vi "诊断标定4.vi"(8 "CAN端口":u16(ring), 9 "设备索引号":u16(ring), 10 "CAN卡类型":u32(ring)=4) -> ()   [LabVIEW 2013] (continued)
                    n1590 = Increment(x=w2571) -> (x+1=w2730:i32)
                    n1591 = global write "读配置文件全局.vi" "从板个数"(w2571) -> ()
                    n1592 = local write "从板个数"(w2571) -> ()
                    n1593 = Index Array(array=w2594, index #1=4 ("索引"), index #2=5 ("索引"), index #3=6 ("索引")) -> (element #1=w2738:string, element #2=w2737:string, element #3=w2736:string)
                    n1594 = Index Array(array=w2747) -> (element #1=w2745:dbl, element #2=w2744:dbl, element #3=w2743:dbl, element #4=w2742:dbl)  [unwired: 4 in]
                    n1595 = Array Subset(array=w2598, index=w2723, length=w2731) -> (w2715:string[])
                    n1596 = Array Subset(array=w2598, index=w2722, length=w2730) -> (w2713:string[])
                    n1597 = Array Subset(array=w2598, index=w2721, length=w2729) -> (w2712:string[])
                    n1598 = Array Subset(array=w2598, index=w2720, length=w2716) -> (w2711:string[])
                    n1599 = Array Subset(array=w2598, index=w2719, length=20 ("长度")) -> (w2710:string[])
                    n1600 = Array Subset(array=w2598, index=w2718, length=w2717) -> (w2714:string[])
                    n1601 = control-ref of="项目信息2"() -> (w2750:refnum<vi>)
                    n1602 = Insert Into Array(array=w2715, new element #1=w2714, new element #2=w2713, new element #3=w2712, new element #4=w2711, new element #5=w2710) -> (w2568:string[])  [unwired: 1 in]
                    n1603 = property class="Clust (严格)"(reference=w2750) -> (reference out=w2748:refnum<vi>, "Value"=w2749:T8)  [unwired: 1 in, 1 out]
                    n1604 = Array Subset(array=w2602, index=w2723, length=w2716) -> (w2584:string[])
                    n1605 = Array Subset(array=w2602, index=w2722, length=w2716) -> (w2582:string[])
                    n1606 = Array Subset(array=w2602, index=w2721, length=w2716) -> (w2581:string[])
                    n1607 = Array Subset(array=w2602, index=w2720) -> (w2580:string[])  [unwired: 1 in]
                    n1608 = Array Subset(array=w2602, index=w2719, length=w2717) -> (w2579:string[])
                    n1609 = Array Subset(array=w2602, index=w2718, length=w2717) -> (w2583:string[])
                    n1610 = global write "读配置文件全局.vi" "表格输入"(w2568) -> ()
                    n1611 = Bundle(cluster=w2749, "电池额定容量(A)"=w2745, "使用者"=w2735, "电池实际容量(A)"=w2744, "车架(牌)号"=w2737, "配置文件版本"=w2736, "SOH(%)"=w2742, "SOC(%)"=w2743, "产品编号"=w2738) -> (w2569:T8)  [unwired: 1 in]
                    n1612 = Multiply(x=w2571, y=4) -> (x*y=w2575:i32)
                    n1613 = Insert Into Array(array=w2584, new element #1=w2583, new element #2=w2582, new element #3=w2581, new element #4=w2580, new element #5=w2579) -> (w2578:string[])  [unwired: 1 in]
                    n1614 = Add(x=w2575, y=44) -> (x+y=w2573:i32)
                    n1615 = property class="Clust (严格)"(reference=w2748, "Value"=w2569) -> ()  [unwired: 1 in, 2 out]
                    n1616 = global write "读配置文件全局.vi" "项目信息"(w2569) -> ()
                    n1617 = Array Subset(array=w2578, index=0 ("索引"), length=w2573) -> (w2577:string[])
                    n1618 = Build Array(w2577, w2568) -> (w2709:string[][])
                    n1619 = Transpose 2D Array(2D array=w2709) -> (transposed array=w2570:string[][])
                    n1620 = local write "项目信息"(w2570) -> ()
                    n1621 = Array Subset(array=w2595, index=w2627, length=15 ("长度")) -> (w2559:string[])
                    n1622 = Array Subset(array=w2595, index=w2630, length=14 ("长度")) -> (w2635:string[])
                    n1623 = Delete From Array(array=w2559, length=4 ("长度"), index=6 ("索引")) -> (deleted portion=w2621:string[], array with subset deleted=w2620:string[])
                    n1624 = for {
                      tunnel: w2635 -> [w2763] mode=indexing
                      tunnel: [w2762] -> w2634 mode=indexing
                      n1625 = Fract/Exp String To Number(string=w2763) -> (number=w2762:dbl)  [unwired: 3 in, 1 out]
                    }
                    n1626 = for {
                      tunnel: w2620 -> [w2761] mode=indexing
                      tunnel: [w2760] -> w2619 mode=indexing
                      n1627 = Fract/Exp String To Number(string=w2761) -> (number=w2760:dbl)  [unwired: 3 in, 1 out]
                    }
                    n1628 = Array Subset(array=w2595, index=w2639, length=51 ("长度")) -> (w2708:string[])
                    n1629 = for {
                      tunnel: w2708 -> [w2765] mode=indexing
                      tunnel: [w2764] -> w2707 mode=indexing
                      n1630 = Fract/Exp String To Number(string=w2765) -> (number=w2764:dbl)  [unwired: 3 in, 1 out]
                    }
                    n1631 = Index Array(array=w2619) -> (element #1=w2614:dbl, element #2=w2613:dbl, element #3=w2612:dbl, element #4=w2611:dbl, element #5=w2610:dbl, element #6=w2609:dbl, element #7=w2608:dbl, element #8=w2607:dbl, element #9=w2606:dbl, element #10=w2605:dbl, element #11=w2604:dbl)  [unwired: 11 in]
                    n1632 = Delete From Array(array=w2634, length=7 ("长度"), index=0 ("索引")) -> (deleted portion=w2564:dbl[], array with subset deleted=w2632:dbl[])
                    n1633 = Delete From Array(array=w2707, length=17 ("长度"), index=0 ("索引")) -> (deleted portion=w2561:dbl[], array with subset deleted=w2704:dbl[])
                    n1634 = global write "读配置文件全局.vi" "加热控制参数"(w2564) -> ()
                    n1635 = Array To Cluster(array=w2564) -> (cluster=w2633:T23)
                    n1636 = Index Array(array=w2632) -> (element #1=w2592:dbl, element #2=w2591:dbl, element #3=w2590:dbl, element #4=w2589:dbl, element #5=w2588:dbl, element #6=w2587:dbl, element #7=w2586:dbl, element #8=w2585:dbl)  [unwired: 8 in]
                    n1637 = Delete From Array(array=w2704, length=17 ("长度"), index=0 ("索引")) -> (deleted portion=w2560:dbl[], array with subset deleted=w2557:dbl[])
                    n1638 = Index Array(array=w2621) -> (element #1=w2618:string, element #2=w2617:string, element #3=w2615:string, element #4=w2616:string)  [unwired: 4 in]
                    n1639 = local write "加热控制参数"(w2633) -> ()
                    n1640 = global write "读配置文件全局.vi" "一级故障"(w2561) -> ()
                    n1641 = local read "一级故障 5"() -> (w2593:T11)
                    n1642 = global write "读配置文件全局.vi" "二级故障"(w2560) -> ()
                    n1643 = control-ref of="电池信息"() -> (w2625:refnum<vi>)
                    n1644 = property class="Clust (严格)"(reference=w2625) -> (reference out=w2626:refnum<vi>, "Value"=w2624:T12)  [unwired: 1 in, 1 out]
                    n1645 = global write "读配置文件全局.vi" "三级故障"(w2557) -> ()
                    n1646 = Bundle(cluster=w2593, "最大允许单体电压"=w2592, "最大允许总电压"=w2588, "最小允许单体电压"=w2591, "最大允许充电电流"=w2590, "最小允许充电电流"=w2589, "最大允许充电温度"=w2587, "最小允许充电温度"=w2586, "电流步长"=w2585) -> (w2563:T11)
                    n1647 = Bundle(cluster=w2624, "电池串联"=w2614, "电池并联"=w2613, "累计放电总安时"=w2607, "电池包额定容量"=w2612, "电池包额定能量"=w2611, "电池包额定总电压"=w2610, "累计充电总安时"=w2608, "电池充满次数"=w2605, "电池放空次数"=w2606, "电池充电次数"=w2604, "电池生产日期"=w2615, "电池厂家"=w2618, "电池类型"=w2617, "电池包组号"=w2616, "实际容量"=w2609) -> (w2558:T12)  [unwired: 2 in]
                    n1648 = Cluster To Array(cluster=w2563) -> (array=w2562:dbl[])
                    n1649 = local write "一级故障 5"(w2563) -> ()
                    n1650 = global write "读配置文件全局.vi" "充电控制参数"(w2562) -> ()
                    n1651 = property class="Clust (严格)"(reference=w2626, "Value"=w2558) -> ()  [unwired: 1 in, 2 out]
                    n1652 = Index Array(array=w2561) -> (element #1=w2697:dbl, element #2=w2696:dbl, element #3=w2695:dbl, element #4=w2694:dbl, element #5=w2693:dbl, element #6=w2692:dbl, element #7=w2691:dbl, element #8=w2690:dbl, element #9=w2689:dbl, element #10=w2688:dbl, element #11=w2687:dbl, element #12=w2686:dbl, element #13=w2685:dbl, element #14=w2684:dbl, element #15=w2683:dbl, element #16=w2682:dbl, element #17=w2681:dbl)  [unwired: 17 in]
                    n1653 = global write "读配置文件全局.vi" "电池信息"(w2558) -> ()
                    n1654 = Index Array(array=w2560) -> (element #1=w2664:dbl, element #2=w2665:dbl, element #3=w2666:dbl, element #4=w2667:dbl, element #5=w2668:dbl, element #6=w2669:dbl, element #7=w2670:dbl, element #8=w2671:dbl, element #9=w2672:dbl, element #10=w2673:dbl, element #11=w2674:dbl, element #12=w2675:dbl, element #13=w2676:dbl, element #14=w2677:dbl, element #15=w2678:dbl, element #16=w2679:dbl, element #17=w2680:dbl)  [unwired: 17 in]
                    n1655 = Index Array(array=w2557) -> (element #1=w2659:dbl, element #2=w2658:dbl, element #3=w2657:dbl, element #4=w2656:dbl, element #5=w2655:dbl, element #6=w2654:dbl, element #7=w2653:dbl, element #8=w2652:dbl, element #9=w2651:dbl, element #10=w2650:dbl, element #11=w2649:dbl, element #12=w2648:dbl, element #13=w2647:dbl, element #14=w2646:dbl, element #15=w2645:dbl, element #16=w2644:dbl, element #17=w2643:dbl)  [unwired: 17 in]
                    n1656 = control-ref of="一级故障 3"() -> (w2642:refnum<vi>)
                    n1657 = control-ref of="一级故障 2"() -> (w2661:refnum<vi>)
                    n1658 = property class="Clust (严格)"(reference=w2661) -> (reference out=w2663:refnum<vi>, "Value"=w2662:T9)  [unwired: 1 in, 1 out]
                    n1659 = property class="Clust (严格)"(reference=w2642) -> (reference out=w2641:refnum<vi>, "Value"=w2660:T9)  [unwired: 1 in, 1 out]
                    n1660 = Bundle(cluster=w2662, "总电压过高"=w2664, "整组电压不均衡"=w2668, "SOC过高"=w2676, "单体电压过高"=w2672, "总电压过低"=w2665, "温度过高"=w2666, "温度过低"=w2667, "单组电压不均衡"=w2669, "整组温度不均衡"=w2670, "单组温度不均衡"=w2671, "单体电压过低"=w2673, "充电电流过高"=w2674, "放电电流过高"=w2675, "SOC过低"=w2677, "内阻过大"=w2678, "极柱温度过高"=w2679, "SOH过低"=w2680) -> (w2566:T9)
                    n1661 = Bundle(cluster=w2660, "总电压过高"=w2659, "整组电压不均衡"=w2655, "SOC过高"=w2647, "单体电压过高"=w2651, "总电压过低"=w2658, "温度过高"=w2657, "温度过低"=w2656, "单组电压不均衡"=w2654, "整组温度不均衡"=w2653, "单组温度不均衡"=w2652, "单体电压过低"=w2650, "充电电流过高"=w2649, "放电电流过高"=w2648, "SOC过低"=w2646, "内阻过大"=w2645, "极柱温度过高"=w2644, "SOH过低"=w2643) -> (w2565:T9)
                    n1662 = control-ref of="一级故障"() -> (w2700:refnum<vi>)
                    n1663 = property class="Clust (严格)"(reference=w2700) -> (reference out=w2698:refnum<vi>, "Value"=w2699:T9)  [unwired: 1 in, 1 out]
                    n1664 = Bundle(cluster=w2699, "总电压过高"=w2697, "整组电压不均衡"=w2693, "SOC过高"=w2685, "单体电压过高"=w2689, "总电压过低"=w2696, "温度过高"=w2695, "温度过低"=w2694, "单组电压不均衡"=w2692, "整组温度不均衡"=w2691, "单组温度不均衡"=w2690, "单体电压过低"=w2688, "充电电流过高"=w2687, "放电电流过高"=w2686, "SOC过低"=w2684, "内阻过大"=w2683, "极柱温度过高"=w2682, "SOH过低"=w2681) -> (w2567:T9)
                    n1665 = property class="Clust (严格)"(reference=w2698, "Value"=w2567) -> ()  [unwired: 1 in, 2 out]
                    n1666 = property class="Clust (严格)"(reference=w2663, "Value"=w2566) -> ()  [unwired: 1 in, 2 out]
                    n1667 = property class="Clust (严格)"(reference=w2641, "Value"=w2565) -> ()  [unwired: 1 in, 2 out]
                  }
                  frame #2 {
                    (unwired) 2 ("长度")
                    w2808 = 1 ("索引")
                    n1668 = call <vilib>:"Get Section Names.vi"("refnum"=w2824) -> ("section names"=w2825:string[], "refnum out"=w2829:T22)  [unwired: 8 in, 1 out]
                    n1669 = local read "从板板号"() -> (w2806:u8)
                    n1670 = Delete From Array(array=w2825, length=2 ("长度"), index=0 ("索引")) -> (array with subset deleted=w2828:string[])  [unwired: 1 out]
                    n1671 = for {
                      tunnel: w2828 -> [w2843] mode=indexing
                      tunnel: w2829 -> [w2844]
                      tunnel: [w2836] -> w2805 mode=indexing
                      tunnel: [w2835] -> w2794
                      n1672 = call <vilib>:"Get Key Names.vi"("section"=w2843, "refnum"=w2844) -> ("key names"=w2835:string[], "refnum out"=w2842:T22)  [unwired: 6 in, 2 out]
                      n1673 = for {
                        tunnel: w2835 -> [w2848] mode=indexing
                        tunnel: w2843 -> [w2847]
                        tunnel: w2842 -> [w2846]
                        tunnel: [w2845] -> w2836 mode=indexing
                        n1674 = call-poly <vilib>:"Read Key.vi"("section"=w2847, "key"=w2848, "refnum"=w2846) -> ("value"=w2845:string)  [unwired: 5 in, 3 out]
                      }
                      n1675 = Index Array(array=w2836, index=0 ("索引")) -> (element=w2839:string)
                      n1676 = local read "输出数组"() -> (w2840:string[][])
                      n1677 = Decimal String To Number(string=w2839) -> (number=w2838:i32)  [unwired: 2 in, 1 out]
                      n1678 = Decrement(x=w2838) -> (x-1=w2834:i32)
                      n1679 = Replace Array Subset(array=w2840, new element=w2836, index (col)=w2834) -> (w2837:string[][])  [unwired: 1 in]
                      n1680 = local write "输出数组"(w2837) -> ()
                    }
                    "key names" <- w2794
                    n1681 = Decrement(x=w2806) -> (x-1=w2823:u8)
                    n1682 = Index Array(array=w2805, index (row)=w2823) -> (element=w2778:string[])  [unwired: 1 in]
                    n1683 = Search 1D Array(1D array=w2794, element="风机开启温度" ("元素")) -> (index of element=w2811:i32)  [unwired: 1 in]
                    n1684 = Search 1D Array(1D array=w2794, element="电压过高一级" ("元素"), start index (0)=w2811) -> (index of element=w2813:i32)
                    n1685 = Decrement(x=w2811) -> (x-1=w2809:i32)
                    n1686 = Array Subset(array=w2778, index=w2808, length=w2809) -> (w2784:string[])
                    n1687 = Array Subset(array=w2778, index=w2813, length=21 ("长度")) -> (w2821:string[])
                    n1688 = Array Subset(array=w2794, index=w2808, length=w2809) -> (w2783:string[])
                    n1689 = Array Subset(array=w2778, index=w2811, length=7 ("长度")) -> (w2815:string[])
                    n1690 = for {
                      tunnel: w2821 -> [w2831] mode=indexing
                      tunnel: [w2830] -> w2822 mode=indexing
                      n1691 = Fract/Exp String To Number(string=w2831) -> (number=w2830:dbl)  [unwired: 3 in, 1 out]
                    }
                    n1692 = for {
                      tunnel: w2815 -> [w2833] mode=indexing
                      tunnel: [w2832] -> w2780 mode=indexing
                      n1693 = Fract/Exp String To Number(string=w2833) -> (number=w2832:dbl)  [unwired: 3 in, 1 out]
                    }
                    n1694 = Index Array(array=w2778, index=0 ("索引")) -> (element=w2776:string)
                    n1695 = Decimal String To Number(string=w2776) -> (number=w2775:i32)  [unwired: 2 in, 1 out]
                    n1696 = Delete From Array(array=w2822, length=7 ("长度"), index=0 ("索引")) -> (deleted portion=w2782:dbl[], array with subset deleted=w2818:dbl[])
                    n1697 = Array To Cluster(array=w2780) -> (cluster=w2804:T23)
                    n1698 = global write "读配置文件全局2.vi" "加热控制参数"(w2780) -> ()
                    n1699 = global write "读配置文件全局2.vi" "从板板号"(w2775) -> ()
                    n1700 = Delete From Array(array=w2818, length=7 ("长度"), index=0 ("索引")) -> (deleted portion=w2773:dbl[], array with subset deleted=w2774:dbl[])
                    n1701 = local write "加热控制参数"(w2804) -> ()
                    n1702 = Array To Cluster(array=w2782) -> (cluster=w2787:T23)
                    n1703 = Array To Cluster(array=w2774) -> (cluster=w2785:T23)
                    n1704 = Array To Cluster(array=w2773) -> (cluster=w2786:T23)
                    n1705 = global write "读配置文件全局2.vi" "三级故障阀值"(w2774) -> ()
                    n1706 = global write "读配置文件全局2.vi" "一级故障阀值"(w2782) -> ()
                    n1707 = global write "读配置文件全局2.vi" "二级故障阀值"(w2773) -> ()
                    n1708 = local write "一级故障 6"(w2787) -> ()
                    n1709 = local write "一级故障 8"(w2785) -> ()
                    n1710 = local write "一级故障 7"(w2786) -> ()
                    n1711 = Search 1D Array(1D array=w2783, element="温度个数" ("元素")) -> (index of element=w2798:i32)  [unwired: 1 in]
                    n1712 = Search 1D Array(1D array=w2783, element="第一个保险通道" ("元素")) -> (index of element=w2797:i32)  [unwired: 1 in]
                    n1713 = Search 1D Array(1D array=w2783, element="电压个数" ("元素")) -> ()  [unwired: 1 in, 1 out]
                    n1714 = Search 1D Array(1D array=w2783, element="第1通道电压个数" ("元素")) -> (index of element=w2796:i32)  [unwired: 1 in]
                    n1715 = Array Subset(array=w2784, length=2 ("长度")) -> (w2792:string[])  [unwired: 1 in]
                    n1716 = Array Subset(array=w2784, index=w2798) -> (w2790:string[])  [unwired: 1 in]
                    n1717 = Array Subset(array=w2784, index=w2797, length=20 ("长度")) -> (w2789:string[])
                    n1718 = Array Subset(array=w2784, index=w2796, length=20 ("长度")) -> (w2791:string[])
                    n1719 = Insert Into Array(array=w2792, new element #1=w2791, new element #2=w2790, new element #3=w2789) -> (w2779:string[])  [unwired: 1 in]
                    n1720 = Build Array(string[] ["电压个数", "电压起始值", "第1通道电压个数", "第2通道电压个数", "第3通道电压个数", "第4通道电压个数", "第5通道电压个数", "第6通道电压个数", "第7通道电压个数", "第8通道电压个数", "第9通道电压个数", "第10通道电压个数", "第11通道电压个数", "第12通道电压个数", "第13通道电压个数", "第14通道电压个数", "第15通道电压个数", "第16通道电压个数", "第17通道电压个数", "第18通道电压个数", "第19通道电压个数", "第20通道电压个数", "温度个数", "温度起始值", "第一个保险通道", "第一个保险位置", "第二个保险通道", "第二个保险位置", "第三个保险通道", "第三个保险位置", "第四个保险通道", "第四个保险位置", "第五个保险通道", "第五个保险位置", "第六个保险通道", "第六个保险位置", "第七个保险通道", "第七个保险位置", "第八个保险通道", "第八个保险位置", "第九个保险通道", "第九个保险位置", "第十个保险通道", "第十个保险位置"], w2779) -> (w2788:string[][])
                    n1721 = global write "读配置文件全局2.vi" "表格"(w2779) -> ()
                    n1722 = Transpose 2D Array(2D array=w2788) -> (transposed array=w2781:string[][])
                    n1723 = local write "项目信息 2"(w2781) -> ()
                  }
                  frame #3 {
                    n1724 = call <vilib>:"Unset Busy.vi"() -> ()  [unwired: 11 in, 1 out]
                    n1725 = Build Array("读取完成") -> (w2852:string[])
                    n1726 = property on="全部写入" class="Bool (严格)"("DisabledEnum"=0) -> ()  [unwired: 2 in, 2 out]
                    n1727 = call "表格编辑.vi"("新元素/子数组"=w2852, "活动单元格:单元格背景色"=u32 6618880, "MCListbox引用句柄"=w2849) -> ()  [unwired: 9 out]
                  }
                }
              }
            }
          }
        }
      }
      frame Error {
      }
    }
  }
  n1728 = while {
    tunnel: w17 -> [w2874]
    tunnel: w16 -> [w2873]
    tunnel: [w2872] -> w15
    tunnel: [w2871] -> w14
    stop <- w2870 stop-if-true
    n1729 = event shown="[33] \"风机继电器\": 值改变" {
      selector: _ -> [_ _ _ _ _ _ _ _ _ _ _ _ _ _ _ _ _ _ _ _ _ _ _ _ _ _ _ _ _ _ _ _ _ _ _ _ _ _ _ _ _ _ _ _ _ _ _ _ _ _ _]
      dyn-events: _ -> [_ _ _ _ _ _ _ _ _ _ _ _ _ _ _ _ _ _ _ _ _ _ _ _ _ _ _ _ _ _ _ _ _ _ _ _ _ _ _ _ _ _ _ _ _ _ _ _ _ _ _]
      timeout: 200 -> [_ _ _ _ _ _ _ _ _ _ _ _ _ _ _ _ _ _ _ _ _ _ _ _ _ _ _ _ _ _ _ _ _ _ _ _ _ _ _ _ _ _ _ _ _ _ _ _ _ _ _]
      tunnel: [_ w2877 w2905 _ _ _ _ _ _ _ _ _ _ _ _ _ _ _ _ _ _ _ _ _ _ _ _ _ _ _ _ _ _ _ _ _ _ _ _ _ _ _ _ _ _ _ _ _ _ _ _] -> w2869
      tunnel: w2874 -> [w2876 w2880 w2904 w2926 w2932 w2938 w2944 w2950 w2956 w2962 w2968 w2974 w2980 w2986 w3002 w3509 w3761 w3786 w3812 w3896 w3969 w3982 w3992 w4035 _ _ w4083 w4149 w4215 w4281 w4347 w4413 w4479 w4546 w4613 w4679 w4745 w4814 w4825 w4863 w4902 w4941 w4980 w5017 w5077 w5115 w5154 w5190 w5263 w5301 w5339]
      tunnel: w2873 -> [w2875 w2879 w2903 w2925 w2931 w2937 w2943 w2949 w2955 w2961 w2967 w2973 w2979 w2985 w3001 w3508 w3760 w3785 w3811 w3895 w3967 w3980 w3991 w4034 _ _ w4082 w4148 w4214 w4280 w4346 w4412 w4478 w4545 w4612 w4678 w4744 w4812 w4824 w4862 w4901 w4940 w4979 w5016 w5076 w5114 w5153 w5189 w5262 w5300 w5338]
      tunnel: [w2876 w2880 w2904 w2926 w2932 w2938 w2944 w2950 w2956 w2962 w2968 w2974 w2980 w2986 w3002 w3509 w3761 w3786 w3812 w3896 w3968 w3981 w3992 w4035 _ _ w4083 w4149 w4215 w4281 w4347 w4413 w4479 w4546 w4613 w4679 w4745 w4813 w4823 w4861 w4900 w4939 w4978 w5017 w5075 w5113 w5152 w5188 w5261 w5299 w5337] -> w2872
      tunnel: [w2875 w2879 w2903 w2925 w2931 w2937 w2943 w2949 w2955 w2961 w2967 w2973 w2979 w2985 w3001 w3508 w3760 w3785 w3811 w3895 w3966 w3979 w3991 w4034 _ _ w4082 w4148 w4214 w4280 w4346 w4412 w4478 w4545 w4612 w4678 w4744 w4811 w4822 w4860 w4899 w4938 w4977 w5016 w5074 w5112 w5151 w5187 w5260 w5298 w5336] -> w2871
      tunnel: [_ _ _ _ _ _ _ _ _ _ _ _ _ _ _ _ _ _ _ _ _ _ _ _ _ _ _ _ _ _ _ _ _ _ _ _ _ _ w4822 w4860 w4899 w4938 w4977 _ w5074 w5112 w5151 w5187 w5260 w5298 w5336] -> w2868
      event Timeout {
        n1730 = event-data() -> ()  [unwired: 3 out]
      }
      event "停止": Value Change {
        n1731 = event-data() -> ("NewVal"=w2878:bool)  [unwired: 5 out]
        n1732 = stacked-sequence {
          tunnel: w2878 -> [w2886 _]
          tunnel: [w2886 _] -> w2877
          frame #0 {
            n1733 = property class="VI"("FP.State"=T24."Hidden" ("前面板窗口:状态")) -> (reference out=w2882:refnum<vi>, error out=w2881:errorcluster)  [unwired: 2 in]
            n1734 = local write "停止"(TRUE ("停止")) -> ()
            n1735 = property class="VI"(reference=w2882, error in=w2881, "Front Panel.Open"=FALSE ("前面板窗口:打开")) -> ()  [unwired: 2 out]
          }
          frame #1 {
            n1736 = disable-structure shown="启用" {
              frame Disabled {
                n1737 = local read "设备索引号"() -> (w2891:u16)
                n1738 = local read "CAN卡类型"() -> (w2892:u32)
                n1739 = local read "CAN端口"() -> (w2890:u16)
                n1740 = Build Array(7) -> (w2887:i32[])
                n1741 = call "transmit-8.6.vi"("can卡类型"=w2892, "设备索引号"=w2891, "CAN端口"=w2890, "ID"=418398080, "Data"=w2887) -> ()  [unwired: 2 in, 13 out]
              }
              frame Enabled {
                w2899 = u8 0 items=["Normal", "Listen Only"] ("工作方式")
                w2898 = u8 1 items=["Dual Filter", "Single Filter"] ("滤波方式")
                n1742 = local read "设备索引号"() -> (w2894:u16)
                n1743 = local read "CAN卡类型"() -> (w2893:u32)
                n1744 = local read "CAN端口"() -> (w2895:u16)
                n1745 = call "CAN_Init-8.6.vi"("CAN卡类型"=w2893, "设备索引号"=w2894, "CAN端口"=w2895, "操作类型"=enum16{"初始化CAN", "关闭CAN"}."初始化CAN", "滤波方式"=w2898, "Accept Code"=u32 0, "簇"=T20 {"打开CAN"=FALSE, "初始化CAN"=TRUE, "开始CAN"=TRUE, "重启"=FALSE, "关闭CAN"=FALSE}, "Mask Code"=u32 4294967295 ("Accept Code"), "工作方式"=w2899, "是否滤波"=FALSE) -> ()  [unwired: 4 in, 6 out]
              }
            }
          }
        }
      }
      event Panel Close? {
        n1746 = event-data() -> ()  [unwired: 5 out]
        n1747 = stacked-sequence {
          tunnel: [w2906 _] -> w2905
          frame #0 {
            w2906 = TRUE ("前面板窗口:打开")
            n1748 = property class="VI"("FP.State"=T24."Hidden" ("前面板窗口:状态")) -> (reference out=w2908:refnum<vi>, error out=w2907:errorcluster)  [unwired: 2 in]
            n1749 = property class="VI"(reference=w2908, error in=w2907, "Front Panel.Open"=FALSE ("前面板窗口:打开")) -> ()  [unwired: 2 out]
            n1750 = local write "停止"(w2906) -> ()
          }
          frame #1 {
            w2914 = u8 0 items=["Normal", "Listen Only"] ("工作方式")
            w2915 = u8 1 items=["Dual Filter", "Single Filter"] ("滤波方式")
            n1751 = local read "设备索引号"() -> (w2919:u16)
            n1752 = local read "CAN卡类型"() -> (w2920:u32)
            n1753 = local read "CAN端口"() -> (w2918:u16)
            n1754 = call "CAN_Init-8.6.vi"("CAN卡类型"=w2920, "设备索引号"=w2919, "CAN端口"=w2918, "操作类型"=enum16{"初始化CAN", "关闭CAN"}."初始化CAN", "滤波方式"=w2915, "Accept Code"=u32 0, "簇"=T20 {"打开CAN"=FALSE, "初始化CAN"=TRUE, "开始CAN"=TRUE, "重启"=FALSE, "关闭CAN"=FALSE}, "Mask Code"=u32 4294967295 ("Accept Code"), "工作方式"=w2914, "是否滤波"=FALSE) -> ()  [unwired: 4 in, 6 out]
          }
        }
        n1755 = event-data("Discard?"=w2905) -> ()  [unwired: 1 in, 1 out]
      }
      event "1": Value Change {
        w2923 = FALSE ("1")
        n1756 = event-data() -> ()  [unwired: 7 out]
        n1757 = local write "主板2"(T7."项目信息" ("主从板")) -> ()
        n1758 = Not(x=w2923) -> (.not. x?=w2922:bool)
        n1759 = local write "1"(w2922) -> ()
        n1760 = local write "1 2"(w2923) -> ()
        n1761 = local write "1 3"(w2923) -> ()
        n1762 = local write "1 4"(w2923) -> ()
        n1763 = local write "1 5"(w2923) -> ()
        n1764 = local write "1 11"(w2923) -> ()
        n1765 = local write "主板选项"("项目信息" ("主板选项")) -> ()
      }
      event "1 2": Value Change {
        w2929 = FALSE ("1")
        n1766 = event-data() -> ()  [unwired: 7 out]
        n1767 = local write "主板2"(T7."一级故障阀值" ("主从板")) -> ()
        n1768 = Not(x=w2929) -> (.not. x?=w2928:bool)
        n1769 = local write "1"(w2929) -> ()
        n1770 = local write "1 2"(w2928) -> ()
        n1771 = local write "1 3"(w2929) -> ()
        n1772 = local write "1 4"(w2929) -> ()
        n1773 = local write "1 5"(w2929) -> ()
        n1774 = local write "1 11"(w2929) -> ()
        n1775 = local write "主板选项"("一级故障阀值" ("主板选项")) -> ()
      }
      event "1 3": Value Change {
        w2935 = FALSE ("1")
        n1776 = event-data() -> ()  [unwired: 7 out]
        n1777 = local write "主板2"(T7."二级故障阀值" ("主从板")) -> ()
        n1778 = Not(x=w2935) -> (.not. x?=w2934:bool)
        n1779 = local write "1"(w2935) -> ()
        n1780 = local write "1 2"(w2935) -> ()
        n1781 = local write "1 3"(w2934) -> ()
        n1782 = local write "1 4"(w2935) -> ()
        n1783 = local write "1 5"(w2935) -> ()
        n1784 = local write "1 11"(w2935) -> ()
        n1785 = local write "主板选项"("二级故障阀值" ("主板选项")) -> ()
      }
      event "1 4": Value Change {
        w2941 = FALSE ("1")
        n1786 = event-data() -> ()  [unwired: 7 out]
        n1787 = local write "主板2"(T7."三级故障阀值" ("主从板")) -> ()
        n1788 = Not(x=w2941) -> (.not. x?=w2940:bool)
        n1789 = local write "1"(w2941) -> ()
        n1790 = local write "1 2"(w2941) -> ()
        n1791 = local write "1 3"(w2941) -> ()
        n1792 = local write "1 4"(w2940) -> ()
        n1793 = local write "1 5"(w2941) -> ()
        n1794 = local write "1 11"(w2941) -> ()
        n1795 = local write "主板选项"("三级故障阀值" ("主板选项")) -> ()
      }
      event "1 5": Value Change {
        w2947 = FALSE ("1")
        n1796 = event-data() -> ()  [unwired: 7 out]
        n1797 = local write "主板2"(T7."控制参数" ("主从板")) -> ()
        n1798 = Not(x=w2947) -> (.not. x?=w2946:bool)
        n1799 = local write "1"(w2947) -> ()
        n1800 = local write "1 2"(w2947) -> ()
        n1801 = local write "1 3"(w2947) -> ()
        n1802 = local write "1 4"(w2947) -> ()
        n1803 = local write "1 5"(w2946) -> ()
        n1804 = local write "1 11"(w2947) -> ()
        n1805 = local write "主板选项"("加热控制参数" ("主板选项")) -> ()
      }
      event "1 11": Value Change {
        w2953 = FALSE ("1")
        n1806 = event-data() -> ()  [unwired: 7 out]
        n1807 = local write "主板2"(T7."电池信息" ("主从板")) -> ()
        n1808 = Not(x=w2953) -> (.not. x?=w2952:bool)
        n1809 = local write "1"(w2953) -> ()
        n1810 = local write "1 2"(w2953) -> ()
        n1811 = local write "1 3"(w2953) -> ()
        n1812 = local write "1 4"(w2953) -> ()
        n1813 = local write "1 5"(w2953) -> ()
        n1814 = local write "1 11"(w2952) -> ()
        n1815 = local write "主板选项"("电池信息" ("主板选项")) -> ()
      }
      event "1 6": Value Change {
        w2959 = FALSE ("1 6")
        n1816 = event-data() -> ()  [unwired: 7 out]
        n1817 = local write "等级 2"(T13."从板信息" ("等级 2")) -> ()
        n1818 = Not(x=w2959) -> (.not. x?=w2958:bool)
        n1819 = local write "1 6"(w2958) -> ()
        n1820 = local write "1 7"(w2959) -> ()
        n1821 = local write "1 8"(w2959) -> ()
        n1822 = local write "1 9"(w2959) -> ()
        n1823 = local write "1 10"(w2959) -> ()
        n1824 = local write "从板选项"("从板信息" ("从板选项")) -> ()
      }
      event "1 7": Value Change {
        w2965 = FALSE ("1 6")
        n1825 = event-data() -> ()  [unwired: 7 out]
        n1826 = local write "等级 2"(T13."一级故障阀值" ("等级 2")) -> ()
        n1827 = Not(x=w2965) -> (.not. x?=w2964:bool)
        n1828 = local write "1 6"(w2965) -> ()
        n1829 = local write "1 7"(w2964) -> ()
        n1830 = local write "1 8"(w2965) -> ()
        n1831 = local write "1 9"(w2965) -> ()
        n1832 = local write "1 10"(w2965) -> ()
        n1833 = local write "从板选项"("一级故障阀值" ("从板选项")) -> ()
      }
      event "1 8": Value Change {
        w2971 = FALSE ("1 6")
        n1834 = event-data() -> ()  [unwired: 7 out]
        n1835 = local write "等级 2"(T13."二级故障阀值" ("等级 2")) -> ()
        n1836 = Not(x=w2971) -> (.not. x?=w2970:bool)
        n1837 = local write "1 6"(w2971) -> ()
        n1838 = local write "1 7"(w2971) -> ()
        n1839 = local write "1 8"(w2970) -> ()
        n1840 = local write "1 9"(w2971) -> ()
        n1841 = local write "1 10"(w2971) -> ()
        n1842 = local write "从板选项"("二级故障阀值" ("从板选项")) -> ()
      }
      event "1 9": Value Change {
        w2977 = FALSE ("1 6")
        n1843 = event-data() -> ()  [unwired: 7 out]
        n1844 = local write "等级 2"(T13."三级故障阀值" ("等级 2")) -> ()
        n1845 = Not(x=w2977) -> (.not. x?=w2976:bool)
        n1846 = local write "1 6"(w2977) -> ()
        n1847 = local write "1 7"(w2977) -> ()
        n1848 = local write "1 8"(w2977) -> ()
        n1849 = local write "1 9"(w2976) -> ()
        n1850 = local write "1 10"(w2977) -> ()
        n1851 = local write "从板选项"("三级故障阀值" ("从板选项")) -> ()
      }
      event "1 10": Value Change {
        w2983 = FALSE ("1 6")
        n1852 = event-data() -> ()  [unwired: 7 out]
        n1853 = local write "等级 2"(T13."快换参数" ("等级 2")) -> ()
        n1854 = Not(x=w2983) -> (.not. x?=w2982:bool)
        n1855 = local write "1 6"(w2983) -> ()
        n1856 = local write "1 7"(w2983) -> ()
        n1857 = local write "1 8"(w2983) -> ()
        n1858 = local write "1 9"(w2983) -> ()
        n1859 = local write "1 10"(w2982) -> ()
        n1860 = local write "从板选项"("快换参数" ("从板选项")) -> ()
      }
      event "主板选项": Mouse Down {
        n1861 = event-data() -> ("CtlRef"=w3000:refnum<vi>)  [unwired: 8 out]
        n1862 = global read "功能码全局.vi" "主板监控2"() -> (w2989:bool[])
        n1863 = property class="Tree (严格)"(reference=w3000) -> ("Value"=w2992:string)  [unwired: 1 in, 2 out]
        n1864 = Index Array(array=w2989, index=6 ("索引")) -> (element=w2987:bool)
        n1865 = case shown="\"SOC过低(3)\", \"SOC过高(3)\", \"SOH过低(3)\", \"充电电流过高(3)\", \"单体电压过低(3)\", \"单体电压过高(3)\", \"单组电压不均衡(3)\", \"单组温度不均衡(3)\", \"放电电流过高(3)\", \"极柱温度过高(3)\", \"内阻过大(3)\", \"三级故障阀值\", \"温度过低(3)\", \"温度过高(3)\", \"整组电压不均衡(3)\", \"整组温度不均衡(3)\", \"总电压过低(3)\", \"总电压过高(3)\"" w2992 {
          tunnel: [T7."项目信息" ("主从板") T7."项目信息" ("主从板") T7."项目信息" ("主从板") T7."项目信息" ("主从板") T7."项目信息" ("主从板") T7."项目信息" ("主从板") T7."项目信息" ("主从板") T7."项目信息" ("主从板") T7."项目信息" ("主从板") T7."项目信息" ("主从板") T7."项目信息" ("主从板") T7."项目信息" ("主从板") T7."项目信息" ("主从板") T7."项目信息" ("主从板") T7."项目信息" ("主从板") T7."二级故障阀值" ("主从板") T7."三级故障阀值" ("主从板") T7."一级故障阀值" ("主从板") T7."控制参数" ("主从板") T7."控制参数" ("主从板") T7."电池信息" ("主从板") T7."电池信息" ("主从板") T7."电池信息" ("主从板") T7."电池信息" ("主从板") T7."电池信息" ("主从板") T7."项目信息" ("主从板")] -> w2999
          tunnel: [w3008 w3014 w3028 w3044 w3084 w3117 w3163 w3213 w3262 w3296 w3309 w3323 w3337 w3351 w3364 w3376 w3389 w3401 w3414 w3427 w3439 w3452 w3465 w3478 w3491 w3495] -> w2998
          tunnel: [w3009 w3015 w3029 w3045 w3085 w3118 w3164 w3214 w3263 w3297 w3310 w3324 w3338 w3352 w3365 w3376 w3389 w3400 w3414 w3427 w3439 w3452 w3465 w3478 w3491 w3496] -> w2997
          tunnel: [w3009 w3015 w3029 w3045 w3085 w3118 w3164 w3214 w3263 w3297 w3310 w3324 w3338 w3352 w3365 w3377 w3389 w3401 w3414 w3427 w3439 w3452 w3465 w3478 w3491 w3496] -> w2996
          tunnel: [w3009 w3015 w3029 w3045 w3085 w3118 w3164 w3214 w3263 w3297 w3310 w3324 w3338 w3352 w3365 w3376 w3388 w3401 w3414 w3427 w3439 w3452 w3465 w3478 w3491 w3496] -> w2995
          tunnel: [w3009 w3015 w3029 w3045 w3085 w3118 w3164 w3214 w3263 w3297 w3310 w3324 w3338 w3352 w3365 w3376 w3389 w3401 w3413 w3426 w3439 w3452 w3465 w3478 w3491 w3496] -> w2994
          tunnel: [w3009 w3015 w3029 w3045 w3085 w3118 w3164 w3214 w3263 w3297 w3310 w3324 w3338 w3352 w3365 w3376 w3389 w3401 w3414 w3427 w3438 w3451 w3464 w3477 w3490 w3496] -> w2993
          tunnel: [w3007 FALSE w3024 w3036 w3076 w3108 w3154 w3205 w3255 w3291 w3304 w3317 w3330 w3344 w3359 w3372 w3384 w3396 w3409 w3421 w3434 w3446 w3459 w3472 w3485 FALSE] -> w2991
          tunnel: [w3007 TRUE w3021 w3035 w3075 w3109 w3155 w3204 w3254 w3290 w3303 w3316 w3331 w3345 w3358 w3371 w3383 w3395 w3408 w3420 w3433 w3445 w3458 w3471 w3484 FALSE] -> w2990
          tunnel: w2987 -> [w3005 _ w3018 w3032 w3071 w3105 w3151 w3201 w3252 w3287 w3300 w3313 w3327 w3341 w3355 w3368 w3380 w3392 w3405 w3417 w3430 w3441 w3455 w3468 w3481 _]
          frame "项目信息" {
            w3007 = TRUE
            w3009 = FALSE
            n1866 = Select(t=0, s=w3005, f=1) -> (s? t:f=w3003:i32)
            n1867 = property on="项目信息" class="Tbl (严格)"("Disabled"=w3003) -> ()  [unwired: 2 in, 2 out]
            n1868 = property on="电池实际容量(A)" class="DigNum (严格)"("Disabled"=w3003) -> ()  [unwired: 2 in, 2 out]
            n1869 = property on="使用者" class="DigNum (严格)"("Disabled"=w3003) -> ()  [unwired: 2 in, 2 out]
            n1870 = property on="SOH(%)" class="DigNum (严格)"("Disabled"=w3003) -> ()  [unwired: 2 in, 2 out]
            n1871 = property on="电池额定容量(A)" class="DigNum (严格)"("Disabled"=w3003) -> ()  [unwired: 2 in, 2 out]
            n1872 = property on="SOC(%)" class="DigNum (严格)"("Disabled"=w3003) -> ()  [unwired: 2 in, 2 out]
            n1873 = property on="系统时钟" class="Str"("Disabled"=w3003) -> ()  [unwired: 2 in, 2 out]
            n1874 = property on="配置文件版本" class="Str"("Disabled"=w3003) -> ()  [unwired: 2 in, 2 out]
            n1875 = property on="车架(牌)号" class="Str"("Disabled"=w3003) -> ()  [unwired: 2 in, 2 out]
            n1876 = property on="产品编号" class="Str"("Disabled"=w3003) -> ()  [unwired: 2 in, 2 out]
            n1877 = Not(x=w3009) -> (.not. x?=w3008:bool)
          }
          frame "校正时钟" {
            w3013 = 2
            w3015 = FALSE
            n1878 = property on="项目信息" class="Tbl (严格)"("Disabled"=w3013) -> ()  [unwired: 2 in, 2 out]
            n1879 = property on="电池实际容量(A)" class="DigNum (严格)"("Disabled"=w3013) -> ()  [unwired: 2 in, 2 out]
            n1880 = property on="使用者" class="DigNum (严格)"("Disabled"=w3013) -> ()  [unwired: 2 in, 2 out]
            n1881 = property on="SOH(%)" class="DigNum (严格)"("Disabled"=w3013) -> ()  [unwired: 2 in, 2 out]
            n1882 = property on="电池额定容量(A)" class="DigNum (严格)"("Disabled"=w3013) -> ()  [unwired: 2 in, 2 out]
            n1883 = property on="SOC(%)" class="DigNum (严格)"("Disabled"=w3013) -> ()  [unwired: 2 in, 2 out]
            n1884 = property on="系统时钟" class="Str"("Disabled"=w3013) -> ()  [unwired: 2 in, 2 out]
            n1885 = property on="配置文件版本" class="Str"("Disabled"=w3013) -> ()  [unwired: 2 in, 2 out]
            n1886 = property on="车架(牌)号" class="Str"("Disabled"=w3013) -> ()  [unwired: 2 in, 2 out]
            n1887 = property on="产品编号" class="Str"("Disabled"=w3013) -> ()  [unwired: 2 in, 2 out]
            n1888 = Not(x=w3015) -> (.not. x?=w3014:bool)
          }
          frame "产品编号" {
            w3027 = 2
            w3029 = FALSE
            n1889 = property on="项目信息" class="Tbl (严格)"("Disabled"=w3027) -> ()  [unwired: 2 in, 2 out]
            n1890 = property on="电池实际容量(A)" class="DigNum (严格)"("Disabled"=w3027) -> ()  [unwired: 2 in, 2 out]
            n1891 = property on="使用者" class="DigNum (严格)"("Disabled"=w3027) -> ()  [unwired: 2 in, 2 out]
            n1892 = property on="SOH(%)" class="DigNum (严格)"("Disabled"=w3027) -> ()  [unwired: 2 in, 2 out]
            n1893 = property on="电池额定容量(A)" class="DigNum (严格)"("Disabled"=w3027) -> ()  [unwired: 2 in, 2 out]
            n1894 = Select(t=0, s=w3018, f=1) -> (s? t:f=w3017:i32)
            n1895 = property on="SOC(%)" class="DigNum (严格)"("Disabled"=w3027) -> ()  [unwired: 2 in, 2 out]
            n1896 = property on="产品编号" class="Str"("Disabled"=w3017) -> ()  [unwired: 2 in, 2 out]
            n1897 = property on="系统时钟" class="Str"("Disabled"=w3027) -> ()  [unwired: 2 in, 2 out]
            n1898 = property on="配置文件版本" class="Str"("Disabled"=w3027) -> ()  [unwired: 2 in, 2 out]
            n1899 = property on="车架(牌)号" class="Str"("Disabled"=w3027) -> ()  [unwired: 2 in, 2 out]
            n1900 = global read "功能码全局.vi" "主板项目信息5"() -> (w3025:bool[])
            n1901 = global read "功能码全局.vi" "主板项目信息6"() -> (w3022:bool[])
            n1902 = Index Array(array=w3025, index=0 ("索引")) -> (element=w3024:bool)
            n1903 = Index Array(array=w3022, index=1 ("索引")) -> (element=w3021:bool)
            n1904 = Not(x=w3029) -> (.not. x?=w3028:bool)
          }
          frame "电压个数" {
            w3043 = 2
            w3045 = FALSE
            n1905 = local read "从板个数"() -> (w3042:dbl)
            n1906 = property on="电池实际容量(A)" class="DigNum (严格)"("Disabled"=w3043) -> ()  [unwired: 2 in, 2 out]
            n1907 = property on="使用者" class="DigNum (严格)"("Disabled"=w3043) -> ()  [unwired: 2 in, 2 out]
            n1908 = property on="SOH(%)" class="DigNum (严格)"("Disabled"=w3043) -> ()  [unwired: 2 in, 2 out]
            n1909 = property on="电池额定容量(A)" class="DigNum (严格)"("Disabled"=w3043) -> ()  [unwired: 2 in, 2 out]
            n1910 = property on="SOC(%)" class="DigNum (严格)"("Disabled"=w3043) -> ()  [unwired: 2 in, 2 out]
            n1911 = property on="系统时钟" class="Str"("Disabled"=w3043) -> ()  [unwired: 2 in, 2 out]
            n1912 = property on="配置文件版本" class="Str"("Disabled"=w3043) -> ()  [unwired: 2 in, 2 out]
            n1913 = property on="车架(牌)号" class="Str"("Disabled"=w3043) -> ()  [unwired: 2 in, 2 out]
            n1914 = property on="产品编号" class="Str"("Disabled"=w3043) -> ()  [unwired: 2 in, 2 out]
            n1915 = Select(t=0, s=w3032, f=1) -> (s? t:f=w3031:i32)
            n1916 = control-ref of="项目信息"() -> (w3041:refnum<vi>)
            n1917 = stacked-sequence {
              tunnel: w3042 -> [_ w3052 w3064]
              tunnel: w3041 -> [w3047 w3051 w3062]
              frame #0 {
                w3048 = 0
                n1918 = Bundle(w3048, w3048) -> (w3050:cluster{i32, i32})  [unwired: 1 out]
                n1919 = property class="Tbl (严格)"(reference=w3047, "Index Values"=w3050) -> (error out=w3049:errorcluster)  [unwired: 1 in, 1 out]
                n1920 = call <vilib>:"Clear Errors.vi"("error in (no error)"=w3049) -> ()  [unwired: 7 out]
              }
              frame #1 {
                n1921 = for {
                  N: 10 -> [_]
                  tunnel: w3051 -> [w3061]
                  tunnel: w3052 -> [w3056]
                  i -> [w3055]
                  n1922 = Compound Arithmetic op=ADD(1.0 ("值"), w3056, w3055) -> (w3058:dbl)
                  n1923 = Bundle(w3058, 0) -> (w3060:cluster{dbl, i32})  [unwired: 1 out]
                  n1924 = property class="Tbl (严格)"(reference=w3061, "Active Cell"=w3060, "Cell BG Color"=u32 16448250) -> ()  [unwired: 1 in, 2 out]
                }
              }
              frame #2 {
                n1925 = Increment(x=w3064) -> (x+1=w3063:dbl)
                n1926 = for {
                  N: w3063 -> [_]
                  tunnel: w3062 -> [w3065]
                  i -> [w3066]
                  n1927 = Bundle(w3066, 0) -> (w3070:cluster{i32, i32})  [unwired: 1 out]
                  n1928 = property class="Tbl (严格)"(reference=w3065, "Active Cell"=w3070, "Cell BG Color"=u32 6618880) -> (error out=w3067:errorcluster)  [unwired: 1 in, 1 out]
                  n1929 = call <vilib>:"Clear Errors.vi"("error in (no error)"=w3067) -> ()  [unwired: 7 out]
                }
              }
            }
            n1930 = property on="项目信息" class="Tbl (严格)"("Disabled"=w3031) -> ()  [unwired: 2 in, 2 out]
            n1931 = global read "功能码全局.vi" "主板项目信息5"() -> (w3039:bool[])
            n1932 = global read "功能码全局.vi" "主板项目信息6"() -> (w3037:bool[])
            n1933 = Index Array(array=w3039, index=1 ("索引")) -> (element=w3036:bool)
            n1934 = Index Array(array=w3037, index=2 ("索引")) -> (element=w3035:bool)
            n1935 = Not(x=w3045) -> (.not. x?=w3044:bool)
          }
          frame "通道电压数" {
            w3083 = 2
            w3085 = FALSE
            n1936 = property on="电池实际容量(A)" class="DigNum (严格)"("Disabled"=w3083) -> ()  [unwired: 2 in, 2 out]
            n1937 = property on="使用者" class="DigNum (严格)"("Disabled"=w3083) -> ()  [unwired: 2 in, 2 out]
            n1938 = property on="SOH(%)" class="DigNum (严格)"("Disabled"=w3083) -> ()  [unwired: 2 in, 2 out]
            n1939 = property on="电池额定容量(A)" class="DigNum (严格)"("Disabled"=w3083) -> ()  [unwired: 2 in, 2 out]
            n1940 = property on="SOC(%)" class="DigNum (严格)"("Disabled"=w3083) -> ()  [unwired: 2 in, 2 out]
            n1941 = local read "从板个数"() -> (w3081:dbl)
            n1942 = property on="系统时钟" class="Str"("Disabled"=w3083) -> ()  [unwired: 2 in, 2 out]
            n1943 = property on="配置文件版本" class="Str"("Disabled"=w3083) -> ()  [unwired: 2 in, 2 out]
            n1944 = property on="车架(牌)号" class="Str"("Disabled"=w3083) -> ()  [unwired: 2 in, 2 out]
            n1945 = property on="产品编号" class="Str"("Disabled"=w3083) -> ()  [unwired: 2 in, 2 out]
            n1946 = control-ref of="项目信息"() -> (w3082:refnum<vi>)
            n1947 = stacked-sequence {
              tunnel: w3082 -> [w3092 w3095]
              tunnel: w3081 -> [w3091 w3094]
              frame #0 {
                n1948 = Compound Arithmetic op=ADD(1.0 ("值"), w3091) -> (w3088:dbl)
                n1949 = Bundle(w3088, 0) -> (w3090:cluster{dbl, i32})  [unwired: 1 out]
                n1950 = property class="Tbl (严格)"(reference=w3092, "Index Values"=w3090) -> ()  [unwired: 1 in, 2 out]
              }
              frame #1 {
                n1951 = for {
                  N: 20 -> [_]
                  tunnel: w3095 -> [w3103]
                  tunnel: w3094 -> [w3098]
                  i -> [w3097]
                  n1952 = Compound Arithmetic op=ADD(1.0 ("值"), w3098, w3097) -> (w3100:dbl)
                  n1953 = Bundle(w3100, 0) -> (w3102:cluster{dbl, i32})  [unwired: 1 out]
                  n1954 = property class="Tbl (严格)"(reference=w3103, "Active Cell"=w3102, "Cell BG Color"=u32 6618880) -> ()  [unwired: 1 in, 2 out]
                }
              }
            }
            n1955 = Select(t=0, s=w3071, f=1) -> (s? t:f=w3072:i32)
            n1956 = property on="项目信息" class="Tbl (严格)"("Disabled"=w3072) -> ()  [unwired: 2 in, 2 out]
            n1957 = global read "功能码全局.vi" "主板项目信息5"() -> (w3079:bool[])
            n1958 = global read "功能码全局.vi" "主板项目信息6"() -> (w3077:bool[])
            n1959 = Index Array(array=w3079, index=2 ("索引")) -> (element=w3076:bool)
            n1960 = Index Array(array=w3077, index=3 ("索引")) -> (element=w3075:bool)
            n1961 = Not(x=w3085) -> (.not. x?=w3084:bool)
          }
          frame "电压起始值" {
            w3116 = 2
            w3118 = FALSE
            n1962 = property on="电池实际容量(A)" class="DigNum (严格)"("Disabled"=w3116) -> ()  [unwired: 2 in, 2 out]
            n1963 = property on="使用者" class="DigNum (严格)"("Disabled"=w3116) -> ()  [unwired: 2 in, 2 out]
            n1964 = property on="SOH(%)" class="DigNum (严格)"("Disabled"=w3116) -> ()  [unwired: 2 in, 2 out]
            n1965 = property on="电池额定容量(A)" class="DigNum (严格)"("Disabled"=w3116) -> ()  [unwired: 2 in, 2 out]
            n1966 = property on="SOC(%)" class="DigNum (严格)"("Disabled"=w3116) -> ()  [unwired: 2 in, 2 out]
            n1967 = local read "从板个数"() -> (w3114:dbl)
            n1968 = property on="系统时钟" class="Str"("Disabled"=w3116) -> ()  [unwired: 2 in, 2 out]
            n1969 = property on="配置文件版本" class="Str"("Disabled"=w3116) -> ()  [unwired: 2 in, 2 out]
            n1970 = property on="车架(牌)号" class="Str"("Disabled"=w3116) -> ()  [unwired: 2 in, 2 out]
            n1971 = property on="产品编号" class="Str"("Disabled"=w3116) -> ()  [unwired: 2 in, 2 out]
            n1972 = control-ref of="项目信息"() -> (w3115:refnum<vi>)
            n1973 = stacked-sequence {
              tunnel: w3115 -> [w3125 w3128 w3141]
              tunnel: w3114 -> [w3124 w3127 w3140]
              frame #0 {
                n1974 = Compound Arithmetic op=ADD(21.0 ("值"), w3124) -> (w3121:dbl)
                n1975 = Bundle(w3121, 0) -> (w3123:cluster{dbl, i32})  [unwired: 1 out]
                n1976 = property class="Tbl (严格)"(reference=w3125, "Index Values"=w3123) -> ()  [unwired: 1 in, 2 out]
              }
              frame #1 {
                n1977 = for {
                  N: 10 -> [_]
                  tunnel: w3128 -> [w3138]
                  tunnel: w3127 -> [w3133]
                  i -> [w3132]
                  n1978 = Multiply(x=w3133, y=2.0) -> (x*y=w3130:dbl)
                  n1979 = Compound Arithmetic op=ADD(21.0 ("值"), w3130, w3132) -> (w3135:dbl)
                  n1980 = Bundle(w3135, 0) -> (w3137:cluster{dbl, i32})  [unwired: 1 out]
                  n1981 = property class="Tbl (严格)"(reference=w3138, "Active Cell"=w3137, "Cell BG Color"=u32 16448250) -> ()  [unwired: 1 in, 2 out]
                }
              }
              frame #2 {
                n1982 = Increment(x=w3140) -> (x+1=w3139:dbl)
                n1983 = for {
                  N: w3139 -> [_]
                  tunnel: w3141 -> [w3149]
                  tunnel: w3140 -> [w3144]
                  i -> [w3143]
                  n1984 = Compound Arithmetic op=ADD(21.0 ("值"), w3144, w3143) -> (w3146:dbl)
                  n1985 = Bundle(w3146, 0) -> (w3148:cluster{dbl, i32})  [unwired: 1 out]
                  n1986 = property class="Tbl (严格)"(reference=w3149, "Active Cell"=w3148, "Cell BG Color"=u32 6618880) -> ()  [unwired: 1 in, 2 out]
                }
              }
            }
            n1987 = Select(t=0, s=w3105, f=1) -> (s? t:f=w3104:i32)
            n1988 = property on="项目信息" class="Tbl (严格)"("Disabled"=w3104) -> ()  [unwired: 2 in, 2 out]
            n1989 = global read "功能码全局.vi" "主板项目信息5"() -> (w3112:bool[])
            n1990 = global read "功能码全局.vi" "主板项目信息6"() -> (w3110:bool[])
            n1991 = Index Array(array=w3112, index=3 ("索引")) -> (element=w3108:bool)
            n1992 = Index Array(array=w3110, index=4 ("索引")) -> (element=w3109:bool)
            n1993 = Not(x=w3118) -> (.not. x?=w3117:bool)
          }
          frame "温度个数" {
            w3162 = 2
            w3164 = FALSE
            n1994 = property on="电池实际容量(A)" class="DigNum (严格)"("Disabled"=w3162) -> ()  [unwired: 2 in, 2 out]
            n1995 = property on="使用者" class="DigNum (严格)"("Disabled"=w3162) -> ()  [unwired: 2 in, 2 out]
            n1996 = property on="SOH(%)" class="DigNum (严格)"("Disabled"=w3162) -> ()  [unwired: 2 in, 2 out]
            n1997 = property on="电池额定容量(A)" class="DigNum (严格)"("Disabled"=w3162) -> ()  [unwired: 2 in, 2 out]
            n1998 = property on="SOC(%)" class="DigNum (严格)"("Disabled"=w3162) -> ()  [unwired: 2 in, 2 out]
            n1999 = local read "从板个数"() -> (w3160:dbl)
            n2000 = property on="系统时钟" class="Str"("Disabled"=w3162) -> ()  [unwired: 2 in, 2 out]
            n2001 = property on="配置文件版本" class="Str"("Disabled"=w3162) -> ()  [unwired: 2 in, 2 out]
            n2002 = property on="车架(牌)号" class="Str"("Disabled"=w3162) -> ()  [unwired: 2 in, 2 out]
            n2003 = property on="产品编号" class="Str"("Disabled"=w3162) -> ()  [unwired: 2 in, 2 out]
            n2004 = control-ref of="项目信息"() -> (w3161:refnum<vi>)
            n2005 = stacked-sequence {
              tunnel: w3161 -> [w3173 w3176 w3189]
              tunnel: w3160 -> [w3166 w3175 w3188]
              frame #0 {
                n2006 = Multiply(x=w3166, y=2.0) -> (x*y=w3168:dbl)
                n2007 = Compound Arithmetic op=ADD(22.0 ("值"), w3168) -> (w3170:dbl)
                n2008 = Bundle(w3170, 0) -> (w3172:cluster{dbl, i32})  [unwired: 1 out]
                n2009 = property class="Tbl (严格)"(reference=w3173, "Index Values"=w3172) -> ()  [unwired: 1 in, 2 out]
              }
              frame #1 {
                n2010 = for {
                  N: 10 -> [_]
                  tunnel: w3176 -> [w3186]
                  tunnel: w3175 -> [w3181]
                  i -> [w3180]
                  n2011 = Multiply(x=w3181, y=3.0) -> (x*y=w3178:dbl)
                  n2012 = Compound Arithmetic op=ADD(23.0 ("值"), w3178, w3180) -> (w3183:dbl)
                  n2013 = Bundle(w3183, 0) -> (w3185:cluster{dbl, i32})  [unwired: 1 out]
                  n2014 = property class="Tbl (严格)"(reference=w3186, "Active Cell"=w3185, "Cell BG Color"=u32 16448250) -> ()  [unwired: 1 in, 2 out]
                }
              }
              frame #2 {
                n2015 = Increment(x=w3188) -> (x+1=w3187:dbl)
                n2016 = for {
                  N: w3187 -> [_]
                  tunnel: w3189 -> [w3199]
                  tunnel: w3188 -> [w3194]
                  i -> [w3193]
                  n2017 = Multiply(x=2.0, y=w3194) -> (x*y=w3191:dbl)
                  n2018 = Compound Arithmetic op=ADD(22.0 ("值"), w3191, w3193) -> (w3196:dbl)
                  n2019 = Bundle(w3196, 0) -> (w3198:cluster{dbl, i32})  [unwired: 1 out]
                  n2020 = property class="Tbl (严格)"(reference=w3199, "Active Cell"=w3198, "Cell BG Color"=u32 6618880) -> ()  [unwired: 1 in, 2 out]
                }
              }
            }
            n2021 = Select(t=0, s=w3151, f=1) -> (s? t:f=w3150:i32)
            n2022 = property on="项目信息" class="Tbl (严格)"("Disabled"=w3150) -> ()  [unwired: 2 in, 2 out]
            n2023 = global read "功能码全局.vi" "主板项目信息5"() -> (w3158:bool[])
            n2024 = global read "功能码全局.vi" "主板项目信息6"() -> (w3156:bool[])
            n2025 = Index Array(array=w3158, index=4 ("索引")) -> (element=w3154:bool)
            n2026 = Index Array(array=w3156, index=5 ("索引")) -> (element=w3155:bool)
            n2027 = Not(x=w3164) -> (.not. x?=w3163:bool)
          }
          frame "温度起始值" {
            w3212 = 2
            w3214 = FALSE
            n2028 = property on="电池实际容量(A)" class="DigNum (严格)"("Disabled"=w3212) -> ()  [unwired: 2 in, 2 out]
            n2029 = property on="使用者" class="DigNum (严格)"("Disabled"=w3212) -> ()  [unwired: 2 in, 2 out]
            n2030 = property on="SOH(%)" class="DigNum (严格)"("Disabled"=w3212) -> ()  [unwired: 2 in, 2 out]
            n2031 = property on="电池额定容量(A)" class="DigNum (严格)"("Disabled"=w3212) -> ()  [unwired: 2 in, 2 out]
            n2032 = property on="SOC(%)" class="DigNum (严格)"("Disabled"=w3212) -> ()  [unwired: 2 in, 2 out]
            n2033 = local read "从板个数"() -> (w3210:dbl)
            n2034 = property on="系统时钟" class="Str"("Disabled"=w3212) -> ()  [unwired: 2 in, 2 out]
            n2035 = property on="配置文件版本" class="Str"("Disabled"=w3212) -> ()  [unwired: 2 in, 2 out]
            n2036 = property on="车架(牌)号" class="Str"("Disabled"=w3212) -> ()  [unwired: 2 in, 2 out]
            n2037 = property on="产品编号" class="Str"("Disabled"=w3212) -> ()  [unwired: 2 in, 2 out]
            n2038 = control-ref of="项目信息"() -> (w3211:refnum<vi>)
            n2039 = stacked-sequence {
              tunnel: w3211 -> [w3223 w3226 w3239]
              tunnel: w3210 -> [w3216 w3225 w3238]
              frame #0 {
                n2040 = Multiply(x=w3216, y=3.0) -> (x*y=w3218:dbl)
                n2041 = Compound Arithmetic op=ADD(23.0 ("值"), w3218) -> (w3220:dbl)
                n2042 = Bundle(w3220, 0) -> (w3222:cluster{dbl, i32})  [unwired: 1 out]
                n2043 = property class="Tbl (严格)"(reference=w3223, "Index Values"=w3222) -> ()  [unwired: 1 in, 2 out]
              }
              frame #1 {
                n2044 = for {
                  N: 10 -> [_]
                  tunnel: w3226 -> [w3236]
                  tunnel: w3225 -> [w3231]
                  i -> [w3230]
                  n2045 = Multiply(x=4.0, y=w3231) -> (x*y=w3228:dbl)
                  n2046 = Compound Arithmetic op=ADD(24.0 ("值"), w3228, w3230) -> (w3233:dbl)
                  n2047 = Bundle(w3233, 0) -> (w3235:cluster{dbl, i32})  [unwired: 1 out]
                  n2048 = property class="Tbl (严格)"(reference=w3236, "Active Cell"=w3235, "Cell BG Color"=u32 16448250) -> ()  [unwired: 1 in, 2 out]
                }
              }
              frame #2 {
                n2049 = Increment(x=w3238) -> (x+1=w3237:dbl)
                n2050 = for {
                  N: w3237 -> [_]
                  tunnel: w3239 -> [w3249]
                  tunnel: w3238 -> [w3244]
                  i -> [w3243]
                  n2051 = Multiply(x=3.0, y=w3244) -> (x*y=w3241:dbl)
                  n2052 = Compound Arithmetic op=ADD(23.0 ("值"), w3241, w3243) -> (w3246:dbl)
                  n2053 = Bundle(w3246, 0) -> (w3248:cluster{dbl, i32})  [unwired: 1 out]
                  n2054 = property class="Tbl (严格)"(reference=w3249, "Active Cell"=w3248, "Cell BG Color"=u32 6618880) -> ()  [unwired: 1 in, 2 out]
                }
              }
            }
            n2055 = Select(t=0, s=w3201, f=1) -> (s? t:f=w3200:i32)
            n2056 = property on="项目信息" class="Tbl (严格)"("Disabled"=w3200) -> ()  [unwired: 2 in, 2 out]
            n2057 = global read "功能码全局.vi" "主板项目信息5"() -> (w3208:bool[])
            n2058 = global read "功能码全局.vi" "主板项目信息6"() -> (w3206:bool[])
            n2059 = Index Array(array=w3208, index=5 ("索引")) -> (element=w3205:bool)
            n2060 = Index Array(array=w3206, index=6 ("索引")) -> (element=w3204:bool)
            n2061 = Not(x=w3214) -> (.not. x?=w3213:bool)
          }
          frame "保险位置" {
            w3261 = 2
            w3263 = FALSE
            n2062 = property on="电池实际容量(A)" class="DigNum (严格)"("Disabled"=w3261) -> ()  [unwired: 2 in, 2 out]
            n2063 = property on="使用者" class="DigNum (严格)"("Disabled"=w3261) -> ()  [unwired: 2 in, 2 out]
